vi "Clear Items.vi"(8 "error in (no error)":errorcluster, 11 "FSM.Annotation in":refnum<class "FSM.Annotation.lvclass">) -> (0 "error out":errorcluster, 3 "FSM.Annotation out":refnum<class "FSM.Annotation.lvclass">)   [LabVIEW 2015, in "FSM.Annotation.lvclass"]
uses:
  FSM.Annotation.lvclass
  FSM.Annotation.lvclass/FSM.Annotation.ctl
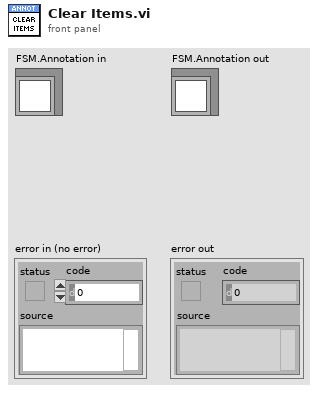
[diagram p1: front panel]
types:
  T1 = cluster{"Name":string, "Style":enum16{"Plain", "On", "Off", "On-Off"}}[]
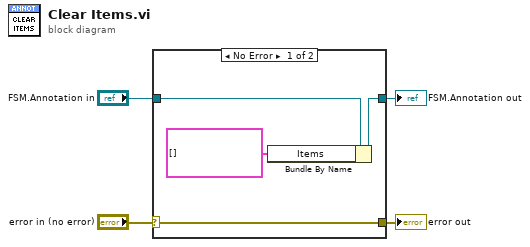
[diagram p0: block diagram]
diagram:
  n1 = case shown="No Error" "error in (no error)" {
    selector: "error in (no error)" -> [w8 w10]
    tunnel: [w8 w10] -> w3
    tunnel: [w5 w9] -> w1
    tunnel: "FSM.Annotation in" -> [w7 w9]
    frame No Error {
      n2 = Bundle By Name(cluster=w7, "Items"=T1 [] ("Serialized.Items")) -> (w5:refnum<class "FSM.Annotation.lvclass">)
    }
    frame Error {
    }
  }
  "error out" <- w3
  "FSM.Annotation out" <- w1
